vi "construct_initialize_hw.vi"(5 "Mode":enum16{"RF", "IF", "BB"}(ring), 11 "error in (no error) 2":errorcluster) -> (4 "command out":T1=enum."configure_rf", 6 "parameters JSON":string, 10 "data out":variant, 14 "Debug info":string, 15 "error out 2":errorcluster)   [LabVIEW 2019, in "mmW_commands.lvlib"]
uses:
  mmW_commands.lvlib
  TypeDefs/_depr_datatypes.ctl
  TypeDefs/commands.ctl
  _depr_initialize_hw.ctl
  <vilib>/addons/_JKI.lib/Serialization/JSON/JKI JSON Serialization.lvlib
panel:
  out "datatype (only for debug)":T2
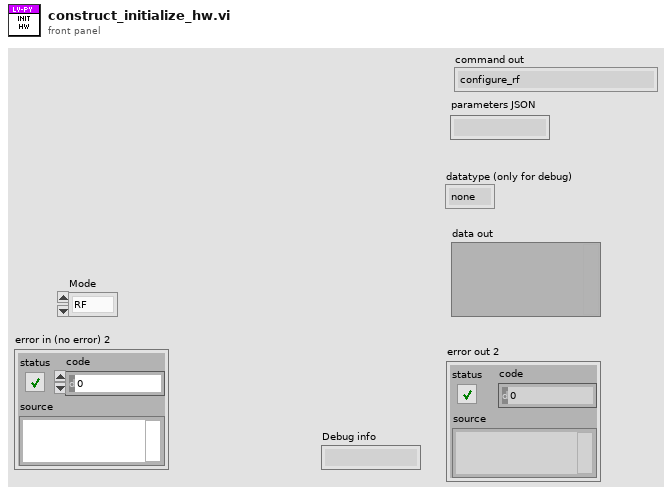
[diagram p1: front panel]
types:
  T1 = typedef "mmW_commands.lvlib/commands.ctl" = enum16{"configure_fs", "configure_rf", "configure_trigger", "equalization_enable", "equalization_start", "lo_sync_enable", "equalization_stop", "get_instrument_status", "get_versions", "initialize_hw", "pop_rx", "set_log_level", "Shutdown", "start", "start_instrument_app", "stop", "trans", "transceive", "trigger_burst", "trigger_sync_enable", "Write TX", "resp_generic", "resp_waveform", "send_trigger", "fetch", "transceive2"}
  T2 = typedef "mmW_commands.lvlib/_depr_datatypes.ctl" = enum16{"none", "float", "string", "CSG_wfm", "DBL_wfm"}
  T3 = typedef "mmW_commands.lvlib/_depr_initialize_hw.ctl" = cluster{"mode":enum16{"RF", "IF", "BB"}, "hwclass":string}
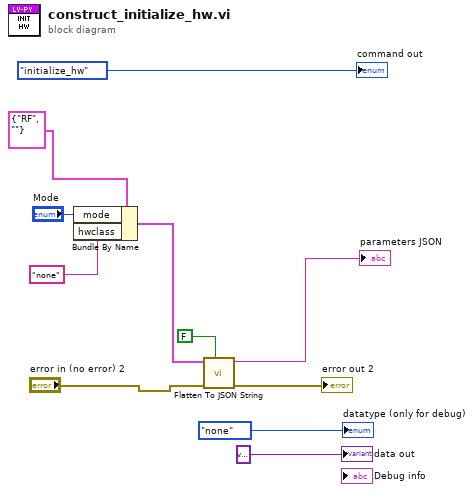
[diagram p0: block diagram]
diagram:
  n1 = Bundle By Name(cluster=T3 {"mode"=enum."RF", "hwclass"=""} ("Cluster"), "mode"="Mode", "hwclass"="none" ("datatype")) -> (w10:T3)
  n2 = call <vilib>:"Flatten To JSON String.vi"("Multiline (T)"=FALSE, "error in (no error)"="error in (no error) 2", "Variant"=w10) -> ("error out"=→"error out 2":errorcluster, "JSON String"=→"parameters JSON":string)  [unwired: 7 in]
  "datatype (only for debug)" <- _depr_datatypes."none" ("datatypes")
  "data out" <- variant
  "command out" <- commands."initialize_hw" ("mmW_instrument_commands")
